vi "Power Analyser FGV Enable.vi"(7 "Enum":T1=enum."WRITE", 11 "Enable":bool=TRUE) -> (3 "Enable Out":bool)   [LabVIEW 2018]
uses:
  Controls/Power Analyser Enum.ctl
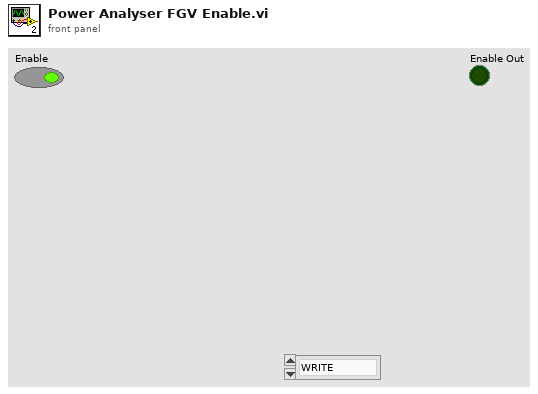
[diagram p1: front panel]
types:
  T1 = typedef "Power Analyser Enum.ctl" = enum16{"READ", "WRITE"}
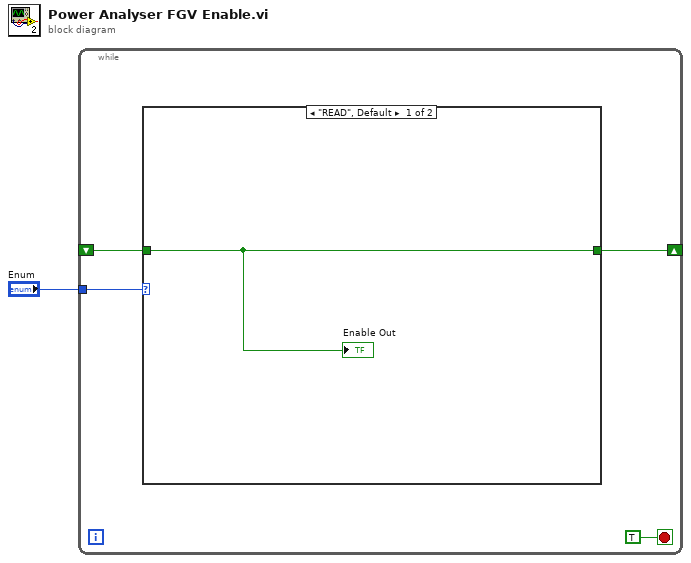
[diagram p0: block diagram]
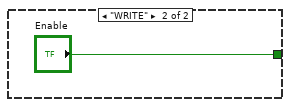
[diagram p2: hidden frame]
diagram:
  n1 = while {
    tunnel: "Enum" -> [w5]
    shift-right: [w3] -> _
    shift-left: _ -> [w2]
    stop <- TRUE stop-if-true
    n2 = case shown="\"READ\", Default" w5 {
      tunnel: [w6 "Enable"] -> w3
      tunnel: w2 -> [w6 _]
      frame "READ", Default {
        "Enable Out" <- w6
      }
      frame "WRITE" {
      }
    }
  }
